vi "03_2.vi"() -> ()   [LabVIEW 2018]
panel:
  out "product":dbl format="%#.0f"
  in  "String":string
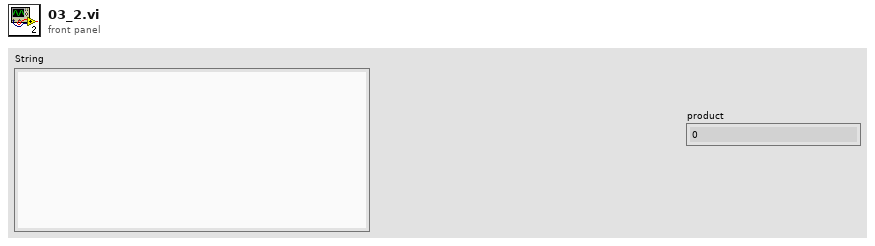
[diagram p1: front panel]
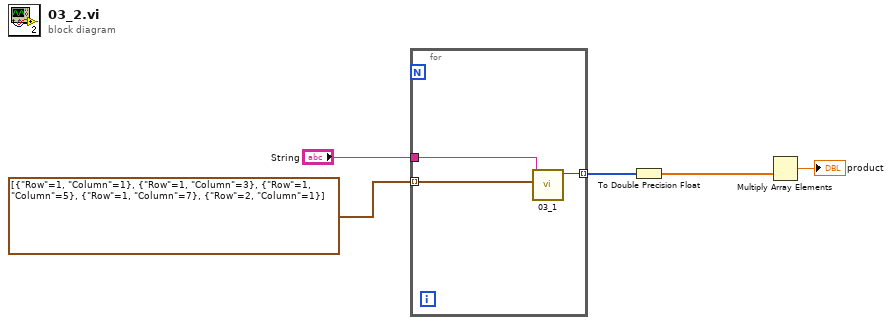
[diagram p0: block diagram]
diagram:
  n1 = for {
    tunnel: [w8] -> w3 mode=indexing
    tunnel: "String" -> [w7]
    tunnel: cluster{"Row":i32, "Column":i32}[] [{"Row"=1, "Column"=1}, {"Row"=1, "Column"=3}, {"Row"=1, "Column"=5}, {"Row"=1, "Column"=7}, {"Row"=2, "Column"=1}] -> [w6] mode=indexing
    n2 = call "03_1.vi"("Increment"=w6, "String"=w7) -> ("size(s)"=w8:i32)  [unwired: 9 in]
  }
  n3 = To Double Precision Float(number=w3) -> (double precision float=w1:dbl[])
  n4 = Multiply Array Elements(1:w1) -> (0:→"product":dbl)
